vi "calc FFT 4chan.vi"(8 "dt":dbl=1e-06 format="%#_13g", 9 "Unit":T1, 10 "Window":T2=1 items=["Rectangle"=0, "Hanning"=1, "Hamming"=2, "Blackman-Harris"=3, "Exact Blackman"=4, "Blackman"=5, "Flat Top"=6, "4 Term B-Harris "=7, "7 Term B-Harris"=8, "Low Sidelobe"=9, "Blackman Nuttall"=11, "Triangle"=30, "Bartlett-Hanning"=31, "Bohman"=32, "Parzen"=33, "Welch"=34, "Kaiser"=60, "Dolph-Chebyshev"=61, "Gaussian"=62], 11 "data":dbl[][](array[numeric])) -> (3 "Power Spectrum / PSD":cluster{"f0":dbl, "df":dbl, "magnitude":dbl[]}[](array[cluster]) {"magnitude" format="%.2p"; "f0" format="%.2p"; "df" format="%.2p"})   [LabVIEW 2013]
uses:
  <vilib>/Analysis/4window.llb/windowTd.ctl
  controls/power_spectrum_unit.ctl
  <vilib>/measure/maspectr.llb/Power Spectrum and PSD Export Mode.ctl
  <vilib>/measure/maspectr.llb/FFT Power Spectrum and PSD for N Chan (CDB).vi
  <vilib>/measure/NI_MAPro.lvlib
  <vilib>/Analysis/NI_AALPro.lvlib
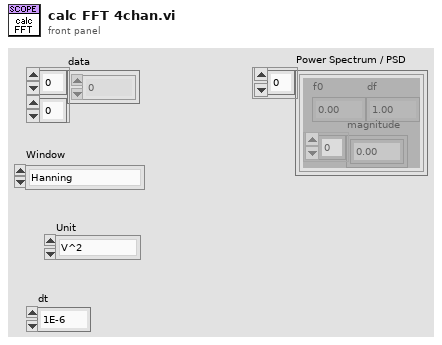
[diagram p1: front panel]
types:
  T1 = typedef "power_spectrum_unit.ctl" = enum16{"V^2", "V", "dBV"}
  T2 = typedef "NI_AALPro.lvlib/windowTd.ctl" = u32
  T3 = typedef "NI_MAPro.lvlib/Power Spectrum and PSD Export Mode.ctl" = u16
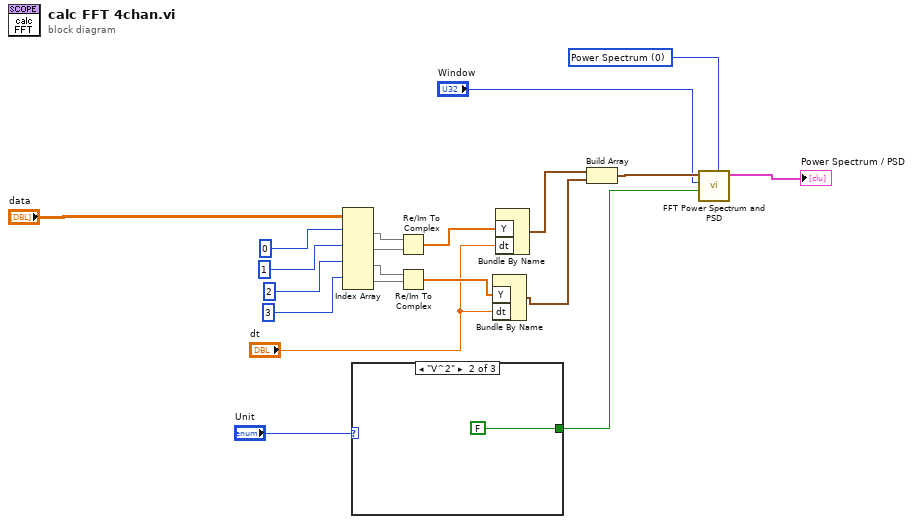
[diagram p0: block diagram]
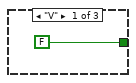
[diagram p2: hidden frame]
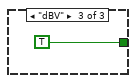
[diagram p3: hidden frame]
diagram:
  w1 = T3 0 items=["Power Spectrum", "Power Spectral Density"] ("export mode")
  n1 = Index Array(array="data", index (row) #1=0 ("index (row)"), index (row) #2=1 ("index (row)"), index (row) #3=2 ("index (row)"), index (row) #4=3 ("index (row)")) -> (element #1=w18:dbl[], element #2=w17:dbl[], element #3=w16:dbl[], element #4=w10:dbl[])  [unwired: 4 in]
  n2 = case shown="\"V^2\"" "Unit" {
    tunnel: [FALSE ("dB On (F)") FALSE ("dB On (F)") TRUE ("dB On (F)")] -> w3
    frame "V" {
    }
    frame "V^2" {
    }
    frame "dBV" {
    }
  }
  n3 = Re/Im To Complex(1:w17, 2:w18) -> (0:w9:cdb[])
  n4 = Re/Im To Complex(1:w10, 2:w16) -> (0:w8:cdb[])
  n5 = Bundle By Name("Y"=w8, "dt"="dt") -> (w7:waveform(cdb))  [unwired: 1 in]
  n6 = Bundle By Name("Y"=w9, "dt"="dt") -> (w20:waveform(cdb))  [unwired: 1 in]
  n7 = Build Array(w20, w7) -> (w19:waveform(cdb)[])
  n8 = call-poly <vilib>:"FFT Power Spectrum and PSD.vi"("export mode"=w1, "dB On (F)"=w3, "window"="Window", "time signals"=w19) -> ("Power Spectrum / PSD"=→"Power Spectrum / PSD":cluster{"f0":dbl, "df":dbl, "magnitude":dbl[]}[])  [unwired: 4 in, 3 out]
